vi "p2.vi"() -> ()   [LabVIEW 2021, in "d15.lvlib"]
uses:
  d15.lvlib
  <vilib>/Analysis/geometry.llb/Point in Polygon Position.ctl
  <vilib>/Analysis/1siggen.llb/Ramp Pattern by Delta.vi
  <vilib>/Analysis/geometry.llb/Point in Polygon (Array).vi
  AOC/AOC.lvlib
  <vilib>/Analysis/NI_AAL_Geometry.lvlib
  <vilib>/Analysis/NI_AALBase.lvlib
panel:
  in  "Example":string="Sensor at x=2, y=18: closest beacon is at x=-2, y=15\nSensor at x=9, y=16: closest beacon is at x=10, y=16\nSensor at x=13, y=2: closest beacon is at x=15, y=3\nSensor at x=12, y=14: closest beacon is at x=10, y=16\nSensor at x=10, y=20: closest beacon is at x=10, y=16\nSensor at x=14, y=17: closest beacon is at x=10, y=16\nSensor at x=8, y=7: closest beacon is at x=2, y=10\nSensor at x=2, y=0: closest beacon is at x=2, y=10\nSensor at x=0, y=11: closest beacon is at x=2, y=10\nSensor at x=20, y=14: closest beacon is at x=25, y=17\nSensor at x=17, y=20: closest beacon is at x=21, y=22\nSensor at x=16, y=7: closest beacon is at x=15, y=3\nSensor at x=14, y=3: closest beacon is at x=15, y=3\nSensor at x=20, y=1: closest beacon is at x=15, y=3"
  in  "Example":bool
  out "Answer":i64=437
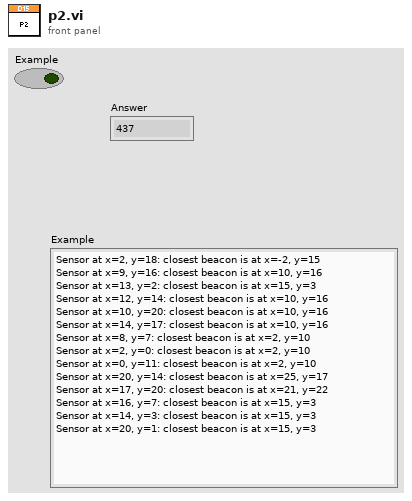
[diagram p1: front panel]
types:
  T1 = typedef "NI_AAL_Geometry.lvlib/Point in Polygon Position.ctl" = u16
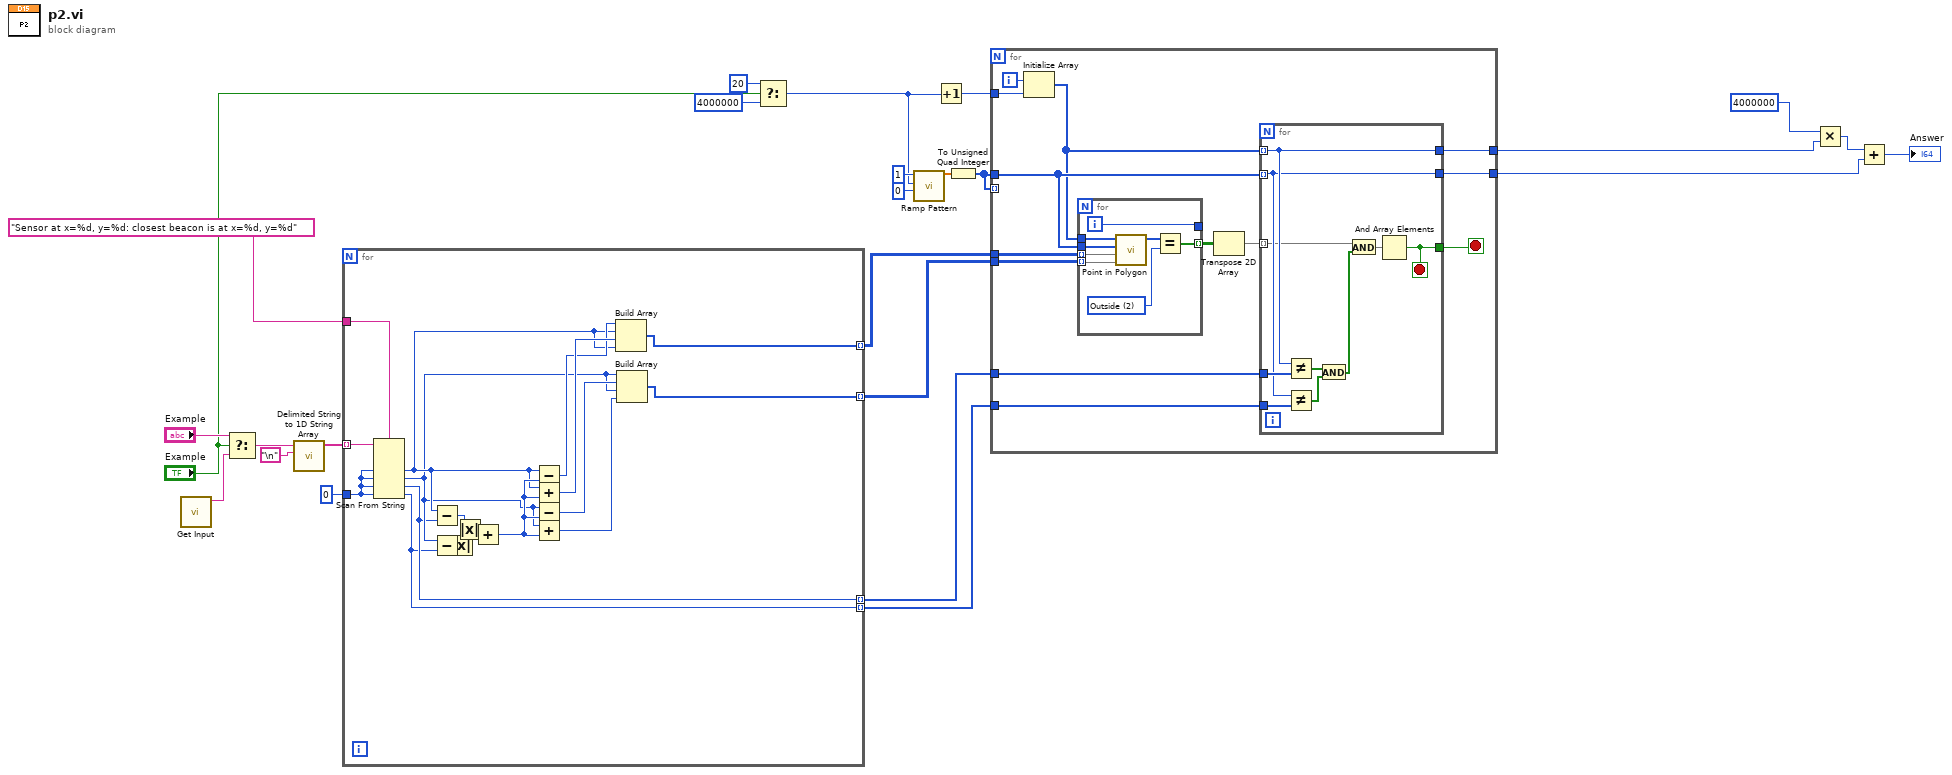
[diagram p0: block diagram]
diagram:
  n1 = call "Get Input.vi"() -> ("Input"=w25:string)  [unwired: 11 in]
  n2 = Select(t="Example", s="Example", f=w25) -> (s? t:f=w24:string)
  n3 = call <vilib>:"Delimited String to 1D String Array.vi"("delimiter"="\n", "delimited string"=w24) -> ("string array"=w19:string[])  [unwired: 9 in]
  n4 = for {
    tunnel: w19 -> [w43] mode=indexing
    tunnel: "Sensor at x=%d, y=%d: closest beacon is at x=%d, y=%d" ("format string") -> [w42]
    tunnel: i64 0 ("default value 1") -> [w41]
    tunnel: [w29] -> w15 mode=indexing
    tunnel: [w28] -> w14 mode=indexing
    tunnel: [w27] -> w13 mode=indexing
    tunnel: [w26] -> w12 mode=indexing
    n5 = Scan From String(format string=w42, input string=w43, default 1=w41, default 2=w41, default 3=w41, default 4=w41) -> (output 1=w31:i64, output 2=w30:i64, output 3=w27:i64, output 4=w26:i64)  [unwired: 2 in, 3 out]
    n6 = Subtract(x=w31, y=w27) -> (x-y=w40:i64)
    n7 = Subtract(x=w30, y=w26) -> (x-y=w39:i64)
    n8 = Absolute Value(x=w39) -> (abs(x)=w37:i64)
    n9 = Absolute Value(x=w40) -> (abs(x)=w38:i64)
    n10 = Add(x=w38, y=w37) -> (x+y=w36:i64)
    n11 = Subtract(x=w31, y=w36) -> (x-y=w33:i64)
    n12 = Add(x=w31, y=w36) -> (x+y=w34:i64)
    n13 = Subtract(x=w30, y=w36) -> (x-y=w35:i64)
    n14 = Add(x=w30, y=w36) -> (x+y=w32:i64)
    n15 = Build Array(w33, w31, w34, w31) -> (w29:i64[])
    n16 = Build Array(w30, w35, w30, w32) -> (w28:i64[])
  }
  n17 = Select(t=20, s="Example", f=4000000) -> (s? t:f=w3:i32)
  n18 = call-poly <vilib>:"Ramp Pattern.vi"("start"=u64 0, "end"=w3, "delta"=u64 1) -> ("Ramp Pattern"=w7:dbl[])  [unwired: 6 in, 2 out]
  n19 = Increment(x=w3) -> (x+1=w4:i32)
  n20 = To Unsigned Quad Integer(1:w7) -> (0:w6:u64[])
  n21 = for {
    tunnel: w15 -> [w56]
    tunnel: w14 -> [w55]
    tunnel: w13 -> [w52]
    tunnel: w12 -> [w51]
    tunnel: [w50] -> w11
    tunnel: [w49] -> w10
    tunnel: w6 -> [_] mode=indexing
    tunnel: w6 -> [w48]
    tunnel: w4 -> [w45]
    i -> [w46]
    stop <- w44 stop-if-true
    n22 = Initialize Array(w46, w45) -> (w47:i32[])
    n23 = for {
      tunnel: w56 -> [w74] mode=indexing
      tunnel: w55 -> [w73] mode=indexing
      tunnel: w47 -> [w69]
      tunnel: w48 -> [w68]
      tunnel: [w70] -> w54 mode=indexing
      tunnel: [w67] -> _
      i -> [w67]
      w71 = T1 2 items=["Inside", "On Boundary", "Outside"] ("y")
      n24 = call-poly <vilib>:"Point in Polygon.vi"("Polygon Y"=w73, "Polygon X"=w74, "Y"=w68, "X"=w69) -> ("Position"=w72:T1[])  [unwired: 6 in, 1 out]
      n25 = Equal?(x=w72, y=w71) -> (x = y?=w70:bool[])
    }
    n26 = Transpose 2D Array(2D array=w54) -> (transposed array=w53:bool[][])
    n27 = for {
      tunnel: w53 -> [w58] mode=indexing
      tunnel: w47 -> [w64] mode=indexing
      tunnel: w48 -> [w61] mode=indexing
      tunnel: [w64] -> w50
      tunnel: [w61] -> w49
      tunnel: w52 -> [w66]
      tunnel: w51 -> [w63]
      tunnel: [w57] -> w44
      stop <- w57 stop-if-true
      n28 = Not Equal?(x=w64, y=w66) -> (x != y?=w65:bool[])
      n29 = Not Equal?(x=w61, y=w63) -> (x != y?=w62:bool[])
      n30 = And(x=w65, y=w62) -> (x .and. y?=w59:bool[])
      n31 = And(x=w58, y=w59) -> (x .and. y?=w60:bool[])
      n32 = And Array Elements(Boolean array=w60) -> (logical AND=w57:bool)
    }
  }
  n33 = Multiply(x=i64 4000000, y=w11) -> (x*y=w18:i64)
  n34 = Add(x=w18, y=w10) -> (x+y=→"Answer":u64)
